vi "M9290A Init and Setup Single Sweep SpecAn.vi"(10 "Ref Level":i32, 11 "VISA resource name":refnum<visa-resource-name>="SpecAn_1") -> (0 "error out":errorcluster, 3 "VISA resource name out":refnum<visa-resource-name>)   [LabVIEW 2015]
uses:
  <instrlib>/Agilent MXA Series/Public/Configure/Configure Frequency (Center Span).vi
  <instrlib>/Agilent MXA Series/Public/Configure/Configure Level (Normal).vi
  <instrlib>/Agilent MXA Series/Public/Configure/Marker/Configure Marker Type (Swept SA).vi
  <instrlib>/Agilent MXA Series/Agilent MXA Series.lvlib
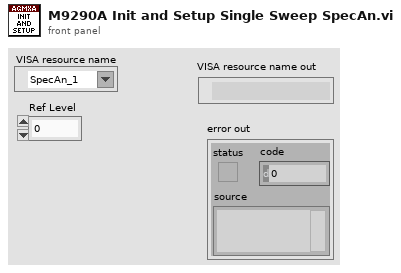
[diagram p1: front panel]
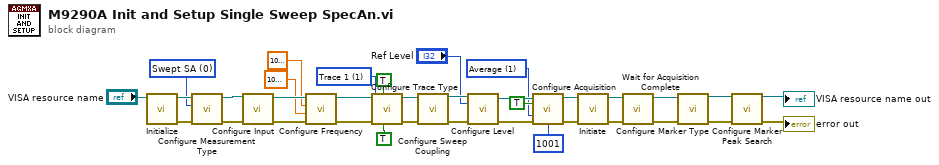
[diagram p0: block diagram]
diagram:
  w1 = 1 items=["Normal", "Average", "Peak", "Sample", "Negative peak"] ("Manual Detector Type (0: Normal)")
  w20 = 1 items=["Trace 1"=1, "Trace 2"=2, "Trace 3"=3, "Trace 4"=4, "Trace 5"=5, "Trace 6"=6] ("Trace Name (1: Trace 1)")
  w27 = 0 items=["Swept SA", "Channel Power", "Occupied Bandwidth", "Power Stat CCDF", "Adjacent Channel Power", "Burst Power", "Spurious Emissions", "Spectrum Emission Mask", "List Sweep", "TOI", "Harmonic"] ("Measurement Type (0: Swept SA)")
  w13 = TRUE ("Enable Continuous Sweep (T: Enable)")
  n1 = call <instrlib>:"Initialize.vi"("VISA resource name"="VISA resource name") -> ("error out"=w29:errorcluster, "VISA resource name out"=w28:refnum<visa-resource-name>)  [unwired: 9 in]
  n2 = call <instrlib>:"Configure Measurement Type.vi"("error in (no error)"=w29, "Measurement Type (0: Swept SA)"=w27, "VISA resource name"=w28) -> ("error out"=w26:errorcluster, "VISA resource name out"=w25:refnum<visa-resource-name>)  [unwired: 7 in]
  n3 = call <instrlib>:"Configure Input.vi"("VISA resource name"=w25, "error in (no error)"=w26) -> ("VISA resource name out"=w24:refnum<visa-resource-name>, "error out"=w23:errorcluster)  [unwired: 12 in]
  n4 = call-poly <instrlib>:"Configure Frequency.vi"("error in (no error)"=w23, "Span (2.65E+10 Hz)"=1000000.0 ("Stop Frequency (2.65E+10 Hz)"), "Center Frequency (1.325E+10 Hz)"=1000000000.0 ("Start Frequency (1E+7 Hz)"), "VISA resource name"=w24) -> ("error out"=w21:errorcluster, "VISA resource name out"=w22:refnum<visa-resource-name>)  [unwired: 6 in]
  n5 = call <instrlib>:"Configure Trace Type.vi"("Enable Trace Display (F: Disable)"=TRUE, "Enable Trace Update (F: Disable)"=TRUE, "error in (no error)"=w21, "Trace Name (1: Trace 1)"=w20, "VISA resource name"=w22) -> ("error out"=w19:errorcluster, "VISA resource name out"=w18:refnum<visa-resource-name>)  [unwired: 5 in]
  n6 = call <instrlib>:"Configure Sweep Coupling.vi"("VISA resource name"=w18, "error in (no error)"=w19) -> ("VISA resource name out"=w17:refnum<visa-resource-name>, "error out"=w16:errorcluster)  [unwired: 12 in]
  n7 = call-poly <instrlib>:"Configure Level.vi"("VISA resource name"=w17, "Reference Level (0 dBm)"="Ref Level", "error in (no error)"=w16) -> ("VISA resource name out"=w14:refnum<visa-resource-name>, "error out"=w15:errorcluster)  [unwired: 11 in]
  n8 = call <instrlib>:"Configure Acquisition.vi"("VISA resource name"=w14, "Enable Continuous Sweep (T: Enable)"=w13, "Auto Detector (T: Enable)"=w13, "Manual Detector Type (0: Normal)"=w1, "error in (no error)"=w15, "Sweep Points (1001)"=1001) -> ("VISA resource name out"=w11:refnum<visa-resource-name>, "error out"=w12:errorcluster)  [unwired: 8 in]
  n9 = call <instrlib>:"Initiate.vi"("error in (no error)"=w12, "VISA resource name"=w11) -> ("error out"=w10:errorcluster, "VISA resource name out"=w9:refnum<visa-resource-name>)  [unwired: 8 in]
  n10 = call <instrlib>:"Wait for Acquisition Complete.vi"("error in (no error)"=w10, "VISA resource name"=w9) -> ("error out"=w7:errorcluster, "VISA resource name out"=w8:refnum<visa-resource-name>)  [unwired: 8 in]
  n11 = call-poly <instrlib>:"Configure Marker Type.vi"("VISA resource name"=w8, "error in (no error)"=w7) -> ("VISA resource name out"=w32:refnum<visa-resource-name>, "error out"=w31:errorcluster)  [unwired: 12 in]
  n12 = call <instrlib>:"Configure Marker Peak Search.vi"("VISA resource name"=w32, "error in (no error)"=w31) -> ("VISA resource name out"=→"VISA resource name out":refnum<visa-resource-name>, "error out"=→"error out":errorcluster)  [unwired: 12 in]
